vi "Actor Create.vi"(9 "Nested Alias":string, 10 "Nested Actor":refnum<class "Actor.lvclass">, 11 "Dev Actor in":refnum<class "Dev Actor.lvclass">) -> (0 "error out":errorcluster, 3 "Dev Actor out":refnum<class "Dev Actor.lvclass">)   [LabVIEW 2021, in "Dev Actor.lvlib" / "Dev Actor.lvclass"]
uses:
  Dev Actor.lvclass
  src/LVCAM/LVCAM/Actor/Actor.lvclass
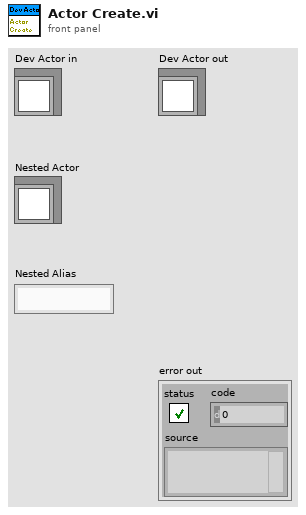
[diagram p1: front panel]
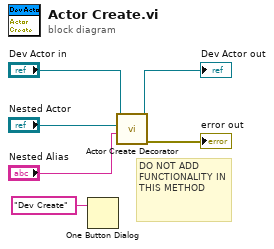
[diagram p0: block diagram]
diagram:
  # "DO NOT ADD FUNCTIONALITY IN THIS METHOD"
  n1 = One Button Dialog(message="Dev Create") -> ()  [unwired: 1 in, 1 out]
  n2 = call "Actor Create Decorator.vi"("Nested Alias"="Nested Alias", "Nested Actor"="Nested Actor", "Dev Actor in"="Dev Actor in") -> ("error out"=→"error out":errorcluster, "Dev Actor out"=→"Dev Actor out":refnum<class "Dev Actor.lvclass">)  [unwired: 7 in]
